vi "Advanced Sweep - Single.vi"() -> ()   [LabVIEW 2016]
uses:
  <instrlib>/Keithley 2600 Series/Public/Channel.ctl
  <instrlib>/Keithley 2600 Series/Keithley 2600 Series.lvlib
panel:
  out "error out":errorcluster
  out "Data Array Out":dbl[](array[numeric])
  in  "Pulse Period (s)":dbl=0.02
  in  "Pulse Width (s)":dbl=0.01
  in  "Pulse Mode (F: Disabled)":bool
  in  "Limit (A)":dbl=0.5
  in  "Stop (V)":dbl
  in  "Start (V)":dbl
  in  "Step Numbers":u32=1
  in  "VISA resource name":refnum<visa-resource-name>
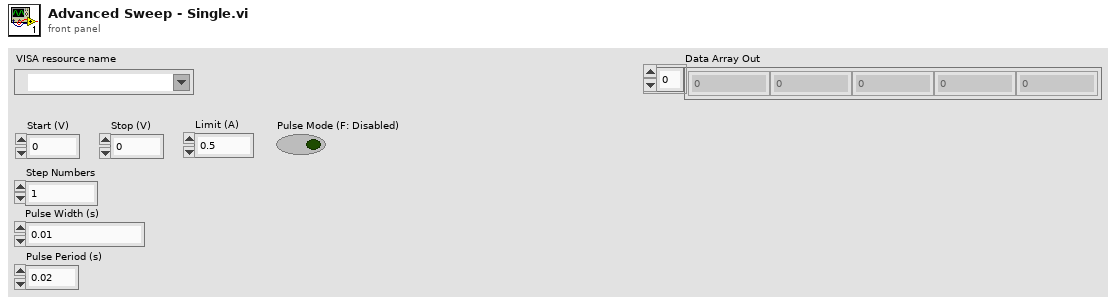
[diagram p1: front panel]
types:
  T1 = enum32{"ASCII", "Real 32", "Real 64", "Single Precision Real", "Double Precision Real"}
  T2 = enum32{"Normal", "Big Endian", "Little Endian", "Network", "Swapped"}
  T3 = enum32{"Digital I/O", "TSP-Link", "LAN", "Software"}
  T4 = enum16{"None/Disconnect", "Digital I/O Trigger", "TSP-Link Trigger", "LAN Trigger", "Blender", "Timer Expired", "Front Panel Trigger", "Software Trigger", "SMU Sweeping", "SMU Armed", "SMU Source Complete", "SMU Measure Complete", "SMU Pulse Complete", "SMU Sweep Complete", "SMU Idle"}
  T5 = enum16{"Current", "Voltage", "IV", "Resistance", "Power"}
  T6 = enum16{"Linear Current", "Linear Voltage", "Logarithimic Current", "Logarithimic Voltage", "List Current", "List Voltage"}
  T7 = typedef "Keithley 2600 Series.lvlib/Channel.ctl" = enum32{"Channel A", "Channel B"}
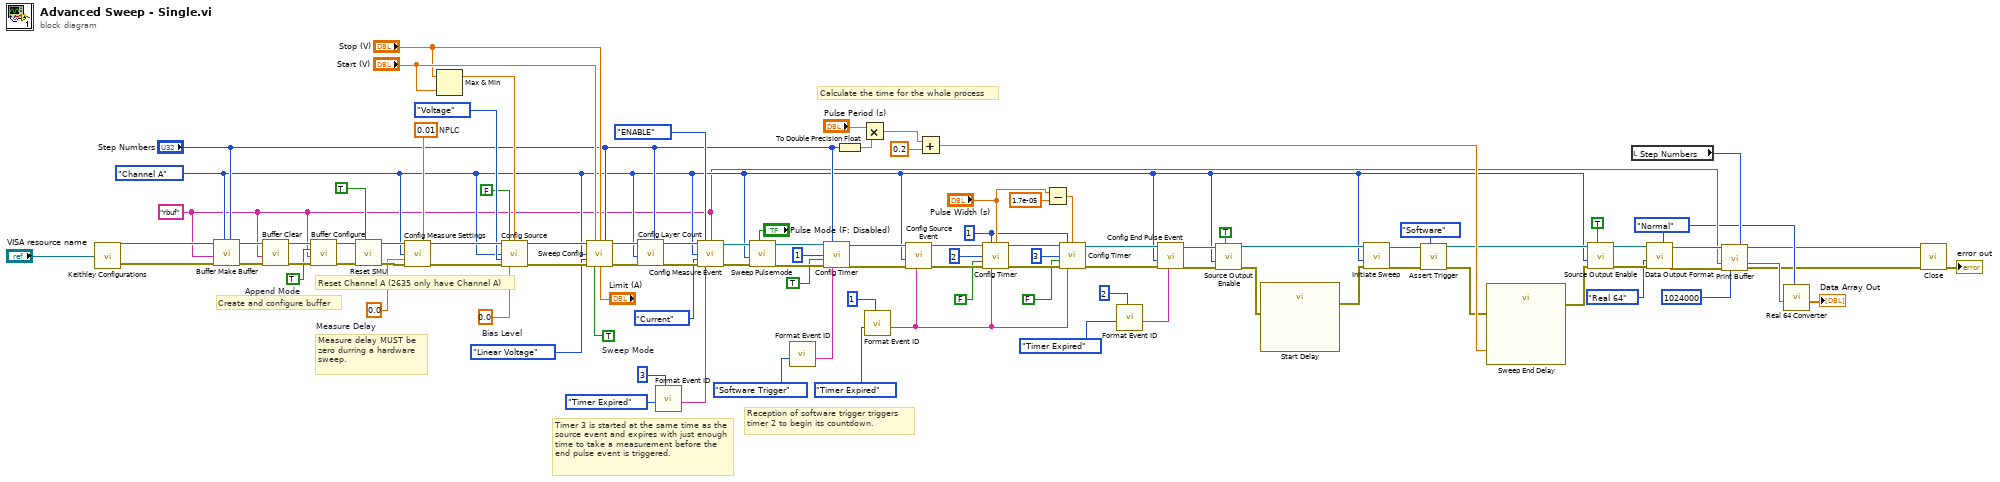
[diagram p0: block diagram]
diagram:
  w5 = T2."Normal" ("Byte Order (Normal)")
  w41 = u32 1 ("Count (1)")
  w78 = TRUE  # Sweep Mode
  w84 = 0.0  # Bias Level
  w88 = 0.01  # NPLC
  w89 = 0.0  # Measure Delay
  w95 = TRUE  # Append Mode
  w9 = "rbuf" ("Buffer Name (buf)")
  w16 = Channel."Channel A" ("Channel (Channel A)")
  # "Calculate the time for the whole process"
  # "Reception of software trigger triggers timer 2 to begin its countdown."
  # "Timer 3 is started at the same time as the source event and expires with just enough time to take a measurement before the end pulse event is triggered."
  # "Measure delay MUST be zero durring a hardware sweep."
  # "Reset Channel A (2635 only have Channel A)"
  # "Create and configure buffer"
  n1 = call "Keithley Configurations.vi"("VISA resource name"="VISA resource name") -> ("VISA resource name out"=w101:refnum<visa-resource-name>, "error out"=w100:errorcluster)
  n2 = call "Buffer Make Buffer.vi"("Capacity (1)"="Step Numbers", "Channel (Channel A)"=w16, "error in (no error)"=w100, "Buffer Name (buf)"=w9, "VISA resource name"=w101) -> ("error out"=w99:errorcluster, "VISA resource name out"=w98:refnum<visa-resource-name>)  [unwired: 3 in, 2 out]
  n3 = call "Buffer Clear.vi"("error in (no error)"=w99, "Buffer Name"=w9, "VISA resource name"=w98) -> ("error out"=w97:errorcluster, "VISA resource name out"=w96:refnum<visa-resource-name>)  [unwired: 6 in, 1 out]
  n4 = call "Buffer Configure.vi"("error in (no error)"=w97, "Buffer Name"=w9, "Append Mode (Off)"=w95, "VISA resource name"=w96) -> ("error out"=w94:errorcluster, "VISA resource name out"=w93:refnum<visa-resource-name>)  [unwired: 5 in, 1 out]
  n5 = call "Reset SMU.vi"("SMU A (No)"=TRUE, "error in (no error)"=w94, "VISA resource name"=w93) -> ("error out"=w90:errorcluster, "VISA resource name out"=w91:refnum<visa-resource-name>)  [unwired: 5 in, 2 out]
  n6 = call "Config Measure Settings.vi"("VISA resource name"=w91, "NPLC (1.000)"=w88, "Channel (Channel A)"=w16, "Measure Delay (0)"=w89, "error in"=w90) -> ("VISA resource name out"=w87:refnum<visa-resource-name>, "error out"=w86:errorcluster)  [unwired: 7 in, 2 out]
  n7 = Max & Min(x="Stop (V)", y="Start (V)") -> (max(x,y)=w82:dbl)  [unwired: 1 out]
  n8 = call "Config Source.vi"("VISA resource name"=w87, "Autorange (On)"=FALSE, "Range (1.000)"=w82, "Channel (Channel A)"=w16, "Function (Current)"=enum32{"Current", "Voltage"}."Voltage", "error in"=w86, "Level (0.000)"=w84) -> ("VISA resource name out"=w81:refnum<visa-resource-name>, "error out"=w80:errorcluster)  [unwired: 5 in, 2 out]
  n9 = call "Sweep Config.vi"("VISA resource name"=w81, "Start Value"="Start (V)", "End Value"="Stop (V)", "Points (1)"="Step Numbers", "Channel (Channel A)"=w16, "Sweep Type"=T6."Linear Voltage", "error in"=w80, "Sweep Mode (F: Disable)"=w78, "Limit (0.1)"="Limit (A)") -> ("VISA resource name out"=w74:refnum<visa-resource-name>, "error out"=w73:errorcluster)  [unwired: 3 in, 2 out]
  n10 = call "Config Layer Count.vi"("Trigger Count (1)"="Step Numbers", "error in"=w73, "Channel (Channel A)"=w16, "VISA resource name"=w74) -> ("error out"=w71:errorcluster, "VISA resource name out"=w72:refnum<visa-resource-name>)  [unwired: 4 in, 2 out]
  n11 = call "Format Event ID.vi"("Event Module # (1)"=u32 3, "Event Type (None)"=T4."Timer Expired") -> ("Event ID"=w66:string)  [unwired: 8 in, 1 out]
  n12 = call "Config Measure Event.vi"("VISA resource name"=w72, "Configure Measurement (Disable)"=enum8{"DISABLE", "ENABLE", "ASYNC"}."ENABLE", "Buffer 1"=w9, "Channel (Channel A)"=w16, "Function (Current)"=T5."Current", "error in"=w71, "Measure Input Event"=w66) -> ("VISA resource name out"=w65:refnum<visa-resource-name>, "error out"=w64:errorcluster)  [unwired: 5 in, 2 out]
  n13 = call "Sweep Pulsemode.vi"("Pulse Mode (F: Disabled)"="Pulse Mode (F: Disabled)", "error in"=w64, "Channel (Channel A)"=w16, "VISA resource name"=w65) -> ("error out"=w61:errorcluster, "VISA resource name out"=w62:refnum<visa-resource-name>)  [unwired: 4 in, 2 out]
  n14 = call "Format Event ID.vi"("Event Type (None)"=T4."Software Trigger") -> ("Event ID"=w57:string)  [unwired: 9 in, 1 out]
  n15 = call "Config Timer.vi"("VISA resource name"=w62, "Count (1)"="Step Numbers", "Timer Number (1)"=u32 1, "Passthrough (Off)"=TRUE, "error in"=w61, "Input Event"=w57) -> ("VISA resource name out"=w56:refnum<visa-resource-name>, "error out"=w55:errorcluster)  [unwired: 6 in, 2 out]
  n16 = To Double Precision Float(number="Step Numbers") -> (double precision float=w25:dbl)
  n17 = Multiply(x="Pulse Period (s)", y=w25) -> (x*y=w22:dbl)
  n18 = call "Format Event ID.vi"("Event Module # (1)"=u32 1, "Event Type (None)"=T4."Timer Expired") -> ("Event ID"=w40:string)  [unwired: 8 in, 1 out]
  n19 = call "Config Source Event.vi"("Input Event"=w40, "error in"=w55, "Channel (Channel A)"=w16, "VISA resource name"=w56) -> ("error out"=w51:errorcluster, "VISA resource name out"=w52:refnum<visa-resource-name>)  [unwired: 4 in, 2 out]
  n20 = Add(x=w22, y=0.2) -> (x+y=w20:dbl)
  n21 = call "Config Timer.vi"("VISA resource name"=w52, "Count (1)"=w41, "Delay (1e-3)"="Pulse Width (s)", "Timer Number (1)"=u32 2, "Passthrough (Off)"=FALSE, "error in"=w51, "Input Event"=w40) -> ("VISA resource name out"=w48:refnum<visa-resource-name>, "error out"=w47:errorcluster)  [unwired: 5 in, 2 out]
  n22 = Subtract(x="Pulse Width (s)", y=1.7e-05) -> (x-y=w42:dbl)
  n23 = call "Config Timer.vi"("VISA resource name"=w48, "Count (1)"=w41, "Delay (1e-3)"=w42, "Timer Number (1)"=u32 3, "Passthrough (Off)"=FALSE, "error in"=w47, "Input Event"=w40) -> ("VISA resource name out"=w39:refnum<visa-resource-name>, "error out"=w38:errorcluster)  [unwired: 5 in, 2 out]
  n24 = call "Format Event ID.vi"("Event Module # (1)"=u32 2, "Event Type (None)"=T4."Timer Expired") -> ("Event ID"=w35:string)  [unwired: 8 in, 1 out]
  n25 = call "Config End Pulse Event.vi"("Input Event"=w35, "error in"=w38, "Channel (Channel A)"=w16, "VISA resource name"=w39) -> ("error out"=w33:errorcluster, "VISA resource name out"=w34:refnum<visa-resource-name>)  [unwired: 4 in, 2 out]
  n26 = call "Source Output Enable.vi"("Output (Off)"=TRUE, "error in (no error)"=w33, "Channel (Channel A)"=w16, "VISA resource name"=w34) -> ("error out"=w31:errorcluster, "VISA resource name out"=w30:refnum<visa-resource-name>)  [unwired: 4 in, 2 out]
  n27 = call "Start Delay"("error in (no error)"=w31) -> ("error out"=w29:errorcluster)  [unwired: 10 in]
  n28 = call "Initiate Sweep.vi"("error in"=w29, "Channel (Channel A)"=w16, "VISA resource name"=w30) -> ("error out"=w27:errorcluster, "VISA resource name out"=w28:refnum<visa-resource-name>)  [unwired: 5 in, 2 out]
  n29 = call "Assert Trigger.vi"("Trigger Type (Digital I/O)"=T3."Software", "error in"=w27, "VISA resource name"=w28) -> ("error out"=w19:errorcluster, "VISA resource name out"=w18:refnum<visa-resource-name>)  [unwired: 5 in, 2 out]
  n30 = call "Sweep End Delay"("error in (no error)"=w19, "Delay Time (s)"=w20) -> ("error out"=w17:errorcluster)  [unwired: 9 in]
  n31 = call "Source Output Enable.vi"("Output (Off)"=TRUE, "error in (no error)"=w17, "Channel (Channel A)"=w16, "VISA resource name"=w18) -> ("error out"=w14:errorcluster, "VISA resource name out"=w13:refnum<visa-resource-name>)  [unwired: 4 in, 2 out]
  n32 = local read "Step Numbers"() -> (w7:u32)
  n33 = call "Data Output Format.vi"("Byte Order (Normal)"=w5, "error in (no error)"=w14, "Data Format (ASCII)"=T1."Real 64", "VISA resource name"=w13) -> ("error out"=w10:errorcluster, "VISA resource name out"=w11:refnum<visa-resource-name>)  [unwired: 4 in, 2 out]
  n34 = call "Print Buffer.vi"("VISA resource name"=w11, "End Index (1)"=w7, "Buffer Name(s)"=w9, "error in (no error)"=w10, "Byte Count (1024)"=u32 1024000) -> ("VISA resource name out"=w3:refnum<visa-resource-name>, "Buffer Data"=w6:string, "error out"=w2:errorcluster)  [unwired: 6 in, 2 out]
  n35 = call "Real 64 Converter.vi"("Byte Order (Normal)"=w5, "Data In"=w6) -> ("Data Array Out"=→"Data Array Out":dbl[])  [unwired: 9 in]
  n36 = call <instrlib>:"Close.vi"("error in (no error)"=w2, "VISA resource name"=w3) -> ("error out"=→"error out":errorcluster)  [unwired: 9 in]
